vi "SubVI Call Translator If Exists.vi"(8 "Error In":errorcluster, 10 "VI Path":path=path "C:/Program Files/National Instruments/LabVIEW 2014/vi.lib/Aledyne-TSXperts/Arduino Compatible Compiler for LabVIEW/addons/Arduino Math/Floor.vi", 11 "SubVI Refnum":refnum<vi>) -> (0 "Error Out":errorcluster, 1 "Defines":string[](array[string]), 2 "Includes":string[](array[string])=["<Arduino.h>", "<math.h>"], 3 "Replaced Code":string="a = floor(v);")   [LabVIEW 2014]
doc: "Run Translator.vi if it's there in same directory as SubVI. If SubVI refnum not providedd it's using VI path control."
panel:
  in  "Output Datatypes":string[](array[string])=["int"]
  in  "Input Datatypes":string[](array[string])=["error", "int"]
  in  "Outputs":string[](array[string])=["a"]
  in  "Inputs":string[](array[string])=["error in", "x"]
  in  "Function Name":string="Arduino Math.lvlib:Floor"
  # "JUST FOR NOW, DEBUGGING"
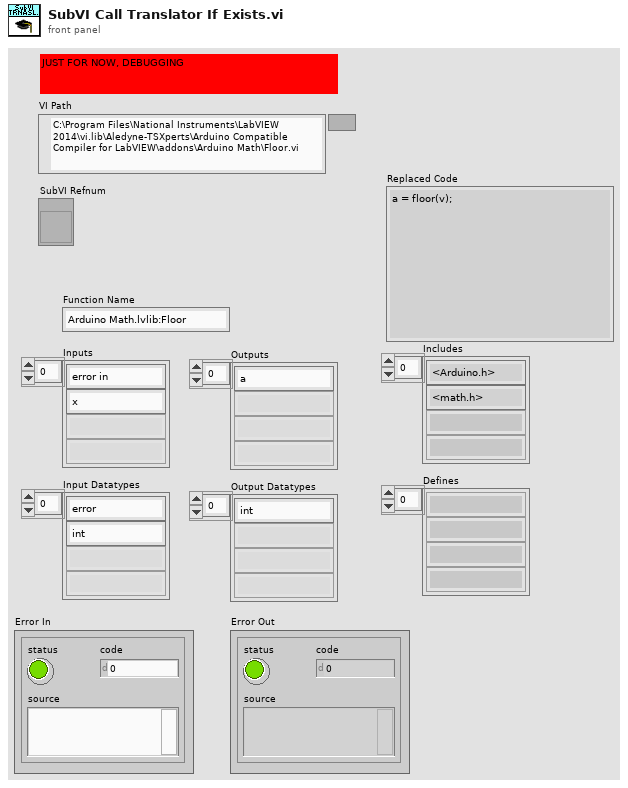
[diagram p1: front panel]
types:
  T1 = cluster{"terminals datatypes":string[][], "terminal\nconnected?":bool[], "terminal captions":string[], "term. count":i32, "terminal\nIsSource?":bool[], "SubVI name":string, "connected\nwires refs.":refnum<vi>[], "coerced dot?":bool[], "terminals[]":refnum<vi>[]}
  T2 = cluster{"wire labels":string[], "wire terminals datatypes":string[][]}
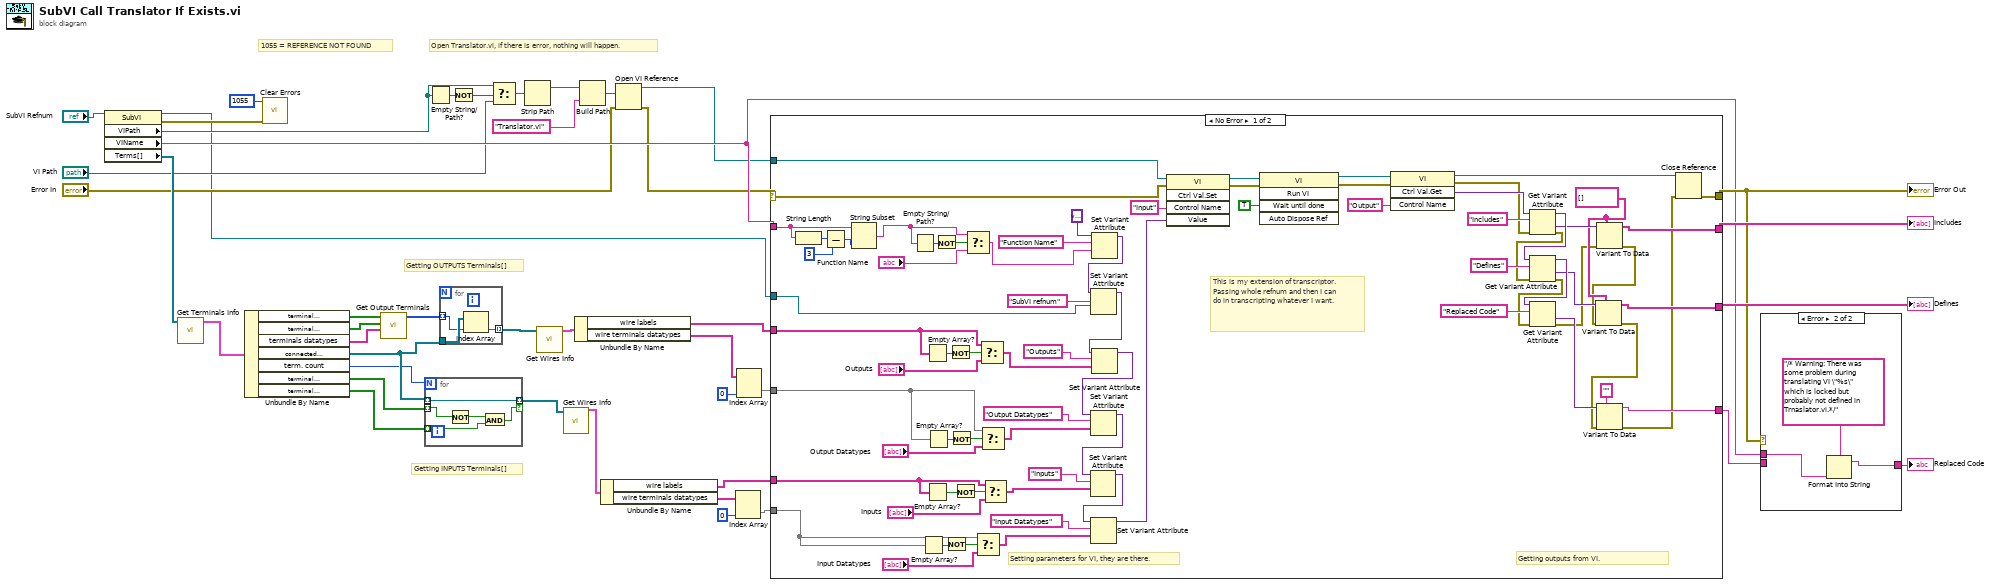
[diagram p0: block diagram]
diagram:
  # "Open Translator.vi, if there is error, nothing will happen."
  # "Getting INPUTS Terminals[]"
  # "Getting OUTPUTS Terminals[]"
  # "1055 = REFERENCE NOT FOUND"
  n1 = property class="SubVI"(reference="SubVI Refnum") -> (reference out=w1:refnum<vi>, error out=w40:errorcluster, "VIPath"=w6:path, "VIName"=w16:string, "Terms[]"=w38:refnum<vi>[])  [unwired: 1 in]
  n2 = call "Get Terminals Info.vi"("Terms[]"=w38) -> ("output cluster"=w37:T1)  [unwired: 9 in, 1 out]
  n3 = Unbundle By Name(w37) -> ("terminal\nconnected?"=w36:bool[], "terminal\nIsSource?"=w35:bool[], "terminals datatypes"=w34:string[][], "connected\nwires refs."=w27:refnum<vi>[], "term. count"=w26:i32, "terminal\nIsSource?"=w15:bool[], "terminal\nconnected?"=w14:bool[])
  n4 = call <vilib>:"Clear Errors.vi"("error in (no error)"=w40, "specific error code to clear (0: all)"=1055) -> ()  [unwired: 4 in, 2 out]
  n5 = call "Get Output Terminals.vi"("terminals datatypes"=w34, "isSource?"=w35, "isConnected?"=w36) -> ("output terminals indexes"=w25:i32[])  [unwired: 8 in]
  n6 = for {
    N: w26 -> [_]
    tunnel: w27 -> [w47] mode=indexing
    tunnel: w15 -> [w48] mode=indexing
    tunnel: [w47] -> w13 mode=indexing if=w44
    tunnel: w14 -> [w45] mode=indexing
    n7 = Not(x=w48) -> (.not. x?=w46:bool)
    n8 = And(x=w46, y=w45) -> (x .and. y?=w44:bool)
  }
  n9 = Empty String/Path?(string/path=w6) -> (empty?=w10:bool)
  n10 = for {
    tunnel: w25 -> [w50] mode=indexing
    tunnel: w27 -> [w51]
    tunnel: [w49] -> w33 mode=indexing
    n11 = Index Array(array=w51, index=w50) -> (element=w49:refnum<vi>)
  }
  n12 = Not(x=w10) -> (.not. x?=w12:bool)
  n13 = Select(t=w6, s=w12, f="VI Path") -> (s? t:f=w11:path)
  n14 = Strip Path(path=w11) -> (stripped path=w7:path)  [unwired: 1 out]
  n15 = call "Get Wires Info.vi"("connected\nwires refs."=w33) -> ("output cluster 2"=w32:T2)  [unwired: 10 in]
  n16 = call "Get Wires Info.vi"("connected\nwires refs."=w13) -> ("output cluster 2"=w24:T2)  [unwired: 10 in]
  n17 = Unbundle By Name(w32) -> ("wire labels"=w31:string[], "wire terminals datatypes"=w30:string[][])
  n18 = Build Path(base path=w7, name or relative path="Translator.vi") -> (appended path=w9:path)
  n19 = Unbundle By Name(w24) -> ("wire labels"=w20:string[], "wire terminals datatypes"=w22:string[][])
  n20 = Open VI Reference(vi path=w9, error in (no error)="Error In") -> (vi reference=w4:refnum<vi>, error out=w2:errorcluster)  [unwired: 4 in]
  n21 = Index Array(array=w22, index (col)=0 ("disabled index (col)")) -> (element=w21:string[])  [unwired: 1 in]
  n22 = Index Array(array=w30, index (col)=0 ("disabled index (col)")) -> (element=w28:string[])  [unwired: 1 in]
  n23 = case shown="No Error" w2 {
    selector: w2 -> [w56 w127]
    tunnel: [w126 w127] -> w19
    tunnel: [w99 _] -> w43
    tunnel: [w98 _] -> w42
    tunnel: [w97 _] -> w17
    tunnel: w16 -> [w61 _]
    tunnel: w31 -> [w90 _]
    tunnel: w28 -> [w77 _]
    tunnel: w21 -> [w78 _]
    tunnel: w20 -> [w70 _]
    tunnel: w4 -> [w57 _]
    tunnel: w1 -> [w52 _]
    frame No Error {
      w101 = string[] [] ("Array - String")
      # "This is my extension of transcriptor. Passing whole refnum and then I can do in transcripting whatever I want."
      # "Getting outputs from VI."
      # "Setting parameters for VI, they are there."
      n24 = String Length(string=w61) -> (length=w60:i32)
      n25 = Subtract(x=w60, y=3) -> (x-y=w59:i32)
      n26 = String Subset(string=w61, length (rest)=w59) -> (substring=w62:string)  [unwired: 1 in]
      n27 = Empty String/Path?(string/path=w62) -> (empty?=w96:bool)
      n28 = Empty Array?(array=w78) -> (empty?=w84:bool)
      n29 = Empty Array?(array=w90) -> (empty?=w89:bool)
      n30 = Empty Array?(array=w70) -> (empty?=w71:bool)
      n31 = Empty Array?(array=w77) -> (empty?=w85:bool)
      n32 = Not(x=w96) -> (.not. x?=w95:bool)
      n33 = Not(x=w84) -> (.not. x?=w83:bool)
      n34 = Not(x=w89) -> (.not. x?=w88:bool)
      n35 = Not(x=w85) -> (.not. x?=w86:bool)
      n36 = Not(x=w71) -> (.not. x?=w72:bool)
      n37 = Select(t=w62, s=w95, f="Function Name") -> (s? t:f=w94:string)
      n38 = Select(t=w78, s=w83, f="Input Datatypes") -> (s? t:f=w82:string[])
      n39 = Select(t=w90, s=w88, f="Outputs") -> (s? t:f=w87:string[])
      n40 = Select(t=w77, s=w86, f="Output Datatypes") -> (s? t:f=w81:string[])
      n41 = Select(t=w70, s=w72, f="Inputs") -> (s? t:f=w74:string[])
      n42 = Set Variant Attribute(Variant=variant ("Value"), name="Function Name", value=w94) -> (Variant out=w55:variant)  [unwired: 1 in, 2 out]
      n43 = Set Variant Attribute(Variant=w55, name="SubVI refnum", value=w52) -> (Variant out=w54:variant)  [unwired: 1 in, 2 out]
      n44 = Set Variant Attribute(Variant=w54, name="Outputs", value=w87) -> (Variant out=w119:variant)  [unwired: 1 in, 2 out]
      n45 = Set Variant Attribute(Variant=w119, name="Output Datatypes", value=w81) -> (Variant out=w76:variant)  [unwired: 1 in, 2 out]
      n46 = Set Variant Attribute(Variant=w76, name="Inputs", value=w74) -> (Variant out=w75:variant)  [unwired: 1 in, 2 out]
      n47 = Set Variant Attribute(Variant=w75, name="Input Datatypes", value=w82) -> (Variant out=w117:variant)  [unwired: 1 in, 2 out]
      n48 = invoke class="VI" method="Ctrl Val.Set"(reference=w57, error in=w56, "Control Name"="Input", "Value"=w117) -> (reference out=w113:refnum<vi>, error out=w112:errorcluster)  [unwired: 1 in, 3 out]
      n49 = invoke class="VI" method="Run VI"(reference=w113, error in=w112, "Wait until done"=TRUE ("Wait Until Done")) -> (reference out=w116:refnum<vi>, error out=w115:errorcluster)  [unwired: 2 in, 3 out]
      n50 = invoke class="VI" method="Ctrl Val.Get"(reference=w116, error in=w115, "Control Name"="Output") -> (reference out=w110:refnum<vi>, error out=w69:errorcluster, "Get Control Value Variant"=w111:variant)  [unwired: 1 in, 1 out]
      n51 = Get Variant Attribute(Variant=w111, name="Includes", error in=w69) -> (duplicate Variant=w106:variant, value=w104:variant, error out=w68:errorcluster)  [unwired: 1 in, 1 out]
      n52 = Get Variant Attribute(Variant=w106, name="Defines", error in=w68) -> (duplicate Variant=w105:variant, value=w103:variant, error out=w67:errorcluster)  [unwired: 1 in, 1 out]
      n53 = Get Variant Attribute(Variant=w105, name="Replaced Code", error in=w67) -> (value=w102:variant, error out=w66:errorcluster)  [unwired: 1 in, 2 out]
      n54 = Variant To Data(error in=w66, type=w101, Variant=w104) -> (data=w99:string[], error out=w65:errorcluster)
      n55 = Variant To Data(error in=w65, type=w101, Variant=w103) -> (data=w98:string[], error out=w64:errorcluster)
      n56 = Variant To Data(error in=w64, type="" ("name"), Variant=w102) -> (data=w97:string, error out=w63:errorcluster)
      n57 = Close Reference(reference=w110, error in (no error)=w63) -> (error out=w126:errorcluster)
    }
    frame Error {
    }
  }
  "Error Out" <- w19
  "Includes" <- w43
  "Defines" <- w42
  n58 = case shown="Error" w19 {
    tunnel: [w128 w129] -> w18
    tunnel: w17 -> [w128 _]
    tunnel: w16 -> [_ w130]
    frame No Error {
    }
    frame Error {
      n59 = Format Into String(format string="/* Warning: There was some problem during translating VI \"%s\" which is locked but probably not defined in Trnaslator.vi.*/", w130) -> (resulting string=w129:string)  [unwired: 2 in, 1 out]
    }
  }
  "Replaced Code" <- w18
